vi "Simulation - RT Plant using so.vi"() -> ()   [LabVIEW 2025]
doc: "This example demonstrates a process simulation for a tank level. The process has added noise, valve deadband, lag, and deadtime. A level controller adjusts the inflow to a tank. An on/off valve serves as a drain that you can click on to operate. This s-valve represents a change in the process loading. You also can switch this VI from automatic control to manual control."
panel:
  in  "Physical Model":bool=TRUE
  in  "Tab Control":enum32{"Introduction", "Operation"}(tab)=enum."Operation"
  out "Flow sensor":bool
  in  "HV-101":bool
  out "tank level":dbl(slide) scale=0.0..100.0 scale format="%#.2g"
  out "Valve":bool
  out "Process Chart":cluster{"Plant Output":dbl, "output":dbl}(graph)
  in  "Stop":bool
  # "Tank Level Control"
  # "Overview: This example demonstrates a process simulation for a tank level.  The process has added noise, valve deadband, lag, and deadtime.  A level controller adjusts the inflow to a tank.  An on/off valve serves as a drain that you can click on to operate.  This s-valve represents a change in the process loading.  You also can switch this VI from automatic control to manual control.\nInstructions:\n1. Run the VI.\n2. Verify the PID controller in closed-loop to track the setpoint.\n3. Change the setpoint to another value and verify the controller tracking the new setpoint.\n4. Apply a disturbance to the system by switching the valve HV 102 (click on the valve symbol). You will see the controller recovering fro the change.\n5. Change PID gains and see if you can improve its performance without going unstable.\n6. Switch to manual mode and see if you can control the level by changing the Valve LVC 101.\n7. Click Stop to stop the VI."
  # "ISA Symbology: The diagram uses the ISA Symbology used for control"
  # "Loop 101"
  # "Level Controller at the control room"
  # "Level Transmitter on the field"
  # "Level Control Valve on the field"
  # "Hand Control Valve on the field"
  # "HV"
  # "102"
  # "LCV"
  # "101"
  # "LIC"
  # "101"
  # "LT"
  # "101"
  # "Slow Leak"
  # "Click to operate"
  # "HV"
  # "102"
  # "LCV"
  # "101"
  # "LIC"
  # "101"
  # "LT"
  # "101"
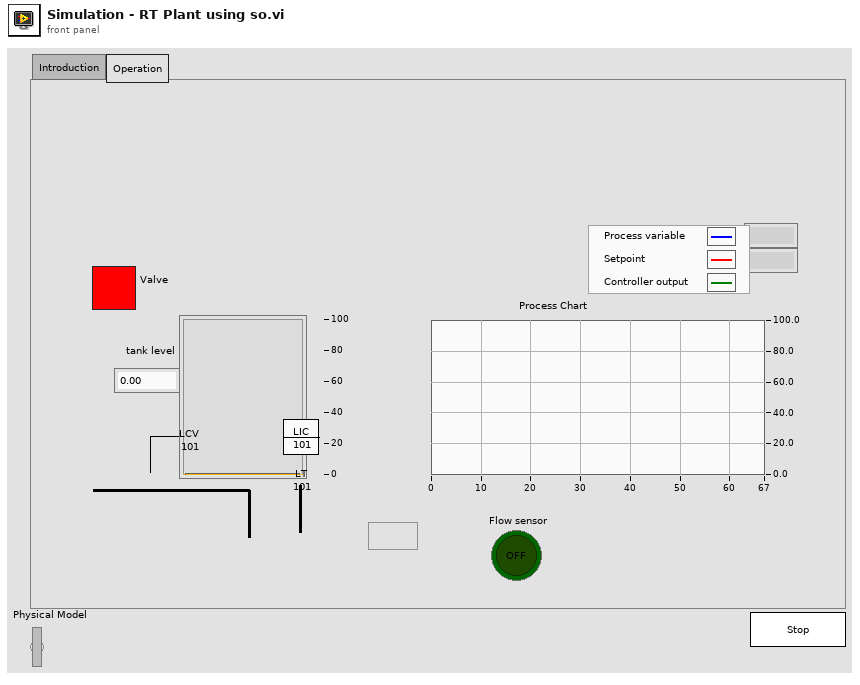
[diagram p1: front panel]
types:
  T1 = cluster{"static gain":dbl, "lag (s)":dbl, "deadtime (s)":dbl, "load":dbl, "deadband":dbl, "sensor noise":dbl, "initial PV":dbl, "plant noise":dbl}
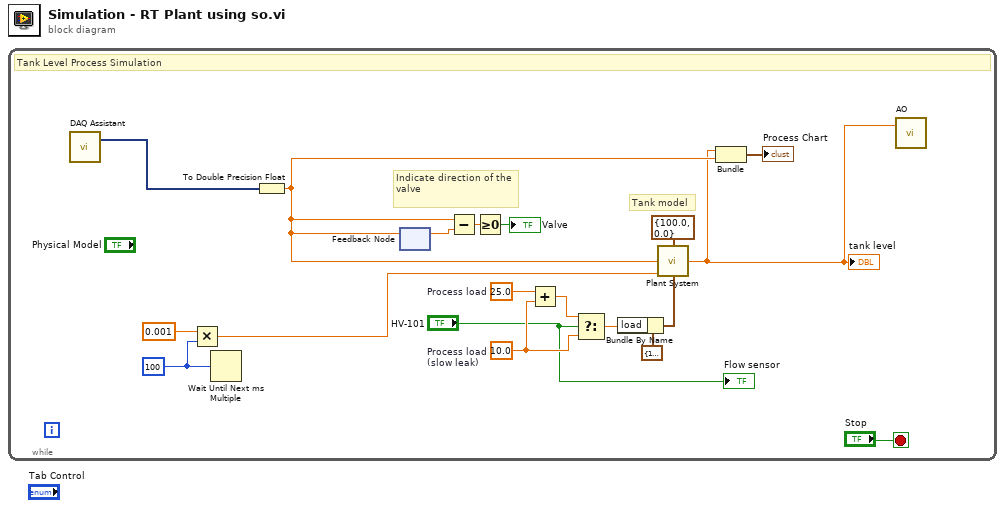
[diagram p0: block diagram]
diagram:
  n1 = while {
    stop <- "Stop" stop-if-true
    w12 = u32 100
    w6 = 25.0  # Process load
    w7 = 10.0  # Process load (slow leak)
    # "Tank model"
    # "Indicate direction of the valve"
    # "Tank Level Process Simulation"
    n2 = call "DAQ Assistant"() -> ("data"=w3:dynamicdata)  [unwired: 17 in, 2 out]
    n3 = Multiply(x=0.001, y=w12) -> (x*y=w11:dbl)
    n4 = Wait Until Next ms Multiple(millisecond multiple=w12) -> ()  [unwired: 1 out]
    n5 = To Double Precision Float(number=w3) -> (double precision float=w2:dbl)
    n6 = feedback-in #1(w2) -> ()
    n7 = feedback #1() -> (w10:dbl)  [unwired: 1 in]
    n8 = Subtract(x=w2, y=w10) -> (x-y=w9:dbl)
    n9 = Greater Or Equal To 0?(x=w9) -> (x >= 0?=→"Valve":bool)
    n10 = Add(x=w6, y=w7) -> (x+y=w5:dbl)
    n11 = Select(t=w5, s="HV-101", f=w7) -> (s? t:f=w15:dbl)
    n12 = Bundle By Name(cluster=T1 {"static gain"=1.5, "lag (s)"=18.0, "deadtime (s)"=1.0, "load"=0.0, "deadband"=1.0, "sensor noise"=0.0, "initial PV"=0.0, "plant noise"=5.0} ("process parameters"), "load"=w15) -> (w14:T1)
    n13 = call "Plant System.vi"("output saturation range"=cluster{"output high":dbl, "output low":dbl} {"output high"=100.0, "output low"=0.0}, "Plant Input"=w2, "dt (s)"=w11, "process parameters"=w14) -> ("Plant Output"=w1:dbl)  [unwired: 11 in]
    "tank level" <- w1
    n14 = Bundle("Plant Output"=w1, w2) -> (→"Process Chart":cluster{"Plant Output":dbl, dbl})  [unwired: 1 in]
    n15 = call "AO"("data"=w1) -> ()  [unwired: 17 in, 2 out]
    "Flow sensor" <- "HV-101"
  }
